vi "Scan URL for Tokens.vi"(1 "URL":string="myDCPwr_Measure_V_0") -> (0 "Tokens":string[](array[string]))   [LabVIEW 2016, in "CS++FgenGui.lvlib" / "CS++FgenGui.lvclass"]
doc: "Scan URL string for tokens."
uses:
  CS++FgenGui.lvclass
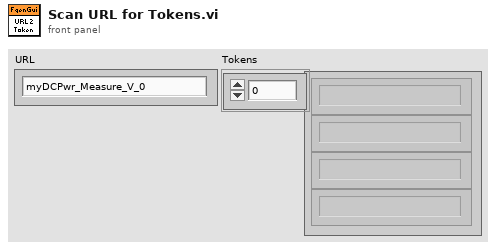
[diagram p1: front panel]
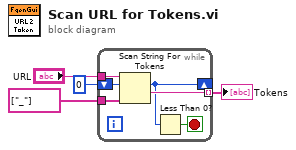
[diagram p0: block diagram]
diagram:
  n1 = while {
    tunnel: "URL" -> [w10]
    tunnel: string[] ["_"] ("delimiters (\\s,\\t,\\r,\\n)") -> [w9]
    shift-right: [w5] -> _
    shift-left: 0 ("offset") -> [w8]
    tunnel: [w7] -> w1 mode=indexing
    stop <- w6 stop-if-true
    n2 = Scan String For Tokens(6:w9, 8:w8, 9:w10) -> (1:w7:string, 2:w5:i32)  [unwired: 3 in, 2 out]
    n3 = Less Than 0?(x=w5) -> (x < 0?=w6:bool)
  }
  "Tokens" <- w1
